vi "AIT 1553 - Parse RT Sysdef Tree Messages.vi"(8 "error in":errorcluster, 9 "RT_Messages":T1[](array[typedef]), 10 "Section Ptr":T3 format="%.0x") -> (0 "error out":errorcluster, 1 "RT_Messages Out":T1[](array[typedef]))   [LabVIEW 2013]
uses:
  <vilib>/NI Veristand/Custom Device API/Custom Device Item Ref.ctl
  Controls/1553_RT_Message.ctl
  Controls/664 -Param.ctl
  Controls and Global/Global.vi
  <vilib>/NI Veristand/Custom Device Tools/Custom Device Utility Library/NI VeriStand - Search for Item by Name.vi
  <vilib>/NI Veristand/Custom Device API/Get Item Property (I32).vi
  <vilib>/NI Veristand/Custom Device API/Get Item Property (Double).vi
  <vilib>/NI Veristand/Custom Device API/Get Item Property (Boolean).vi
  AIT 664 Custom Device.lvlib
  <vilib>/NI Veristand/Custom Device Tools/Custom Device Utility Library/Custom Device Utility Library.lvlib
  <vilib>/NI Veristand/Custom Device API/Custom Device API.lvlib
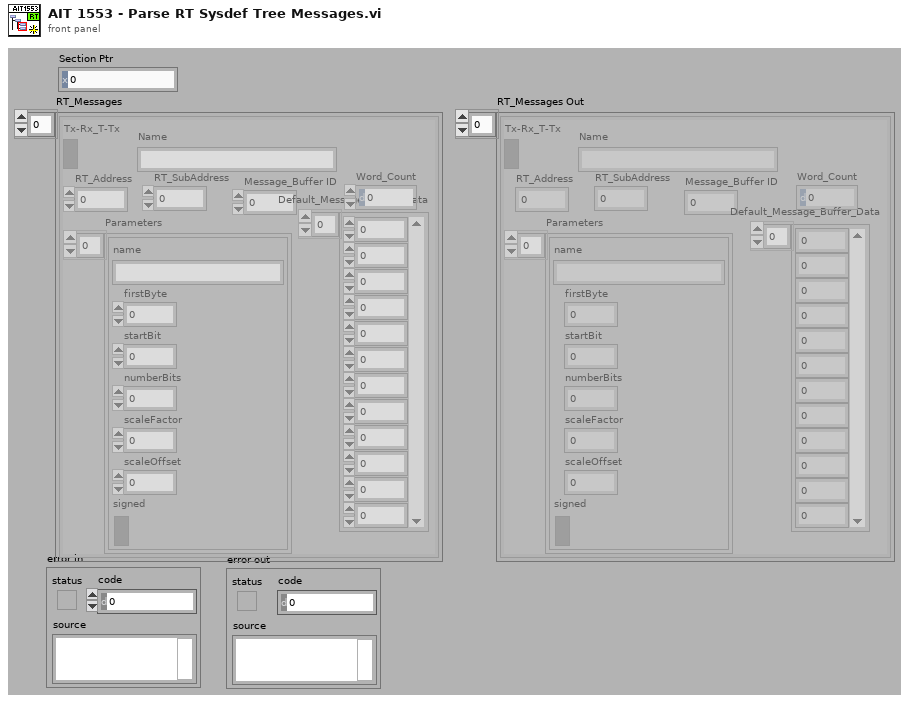
[diagram p1: front panel]
types:
  T1 = typedef "AIT 664 Custom Device.lvlib/1553_RT_Message.ctl" = cluster{"RT_Address":u8, "RT_SubAddress":u8, "Tx-Rx_T-Tx":bool, "Parameters":T2[], "Message_Buffer ID":u16, "Default_Message_Buffer_Data":u16[], "Word_Count":u8, "Name":string}
  T2 = typedef "AIT 664 Custom Device.lvlib/664 -Param.ctl" = cluster{"name":string, "firstByte":i32, "startBit":i32, "numberBits":i32, "scaleFactor":dbl, "scaleOffset":dbl, "signed":bool}
  T3 = typedef "Custom Device API.lvlib/Custom Device Item Ref.ctl" = u64
  T4 = typedef "Custom Device API.lvlib/Custom Device Item Info.ctl" = cluster{"Name":string, "Is Channel":bool, "GUID":string, "Is Waveform":bool}
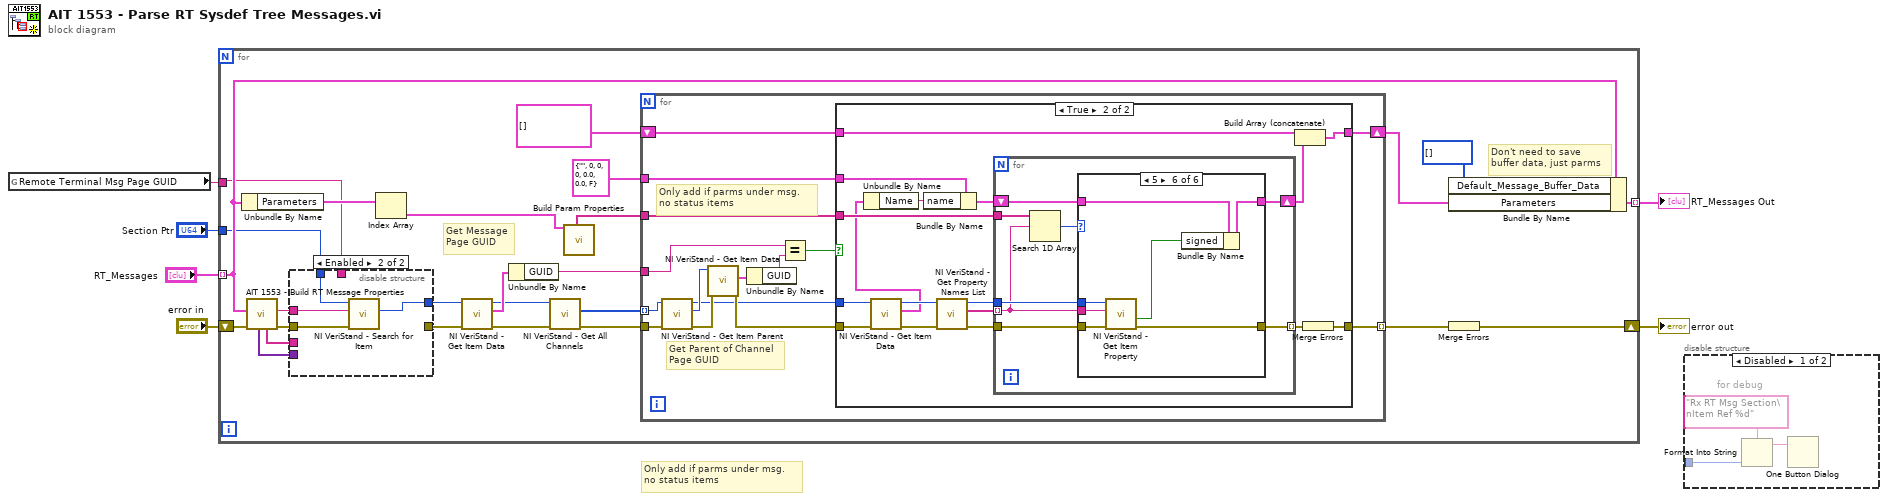
[diagram p0: block diagram]
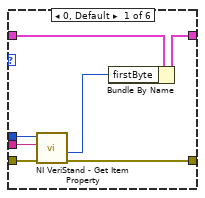
[diagram p4: hidden frame]
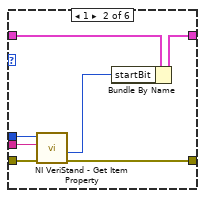
[diagram p5: hidden frame]
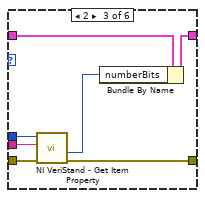
[diagram p6: hidden frame]
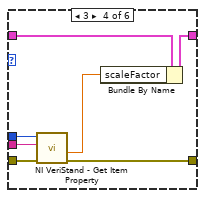
[diagram p7: hidden frame]
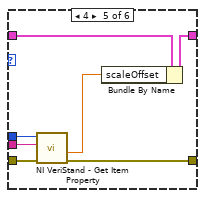
[diagram p8: hidden frame]
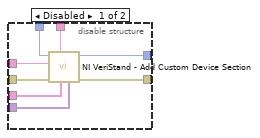
[diagram p9: hidden frame]
diagram:
  # "Only add if parms under msg.\nno status items"
  n1 = global read "Global.vi" "Remote Terminal Msg Page GUID"() -> (w3:string)
  n2 = for {
    shift-right: [w18] -> w6
    shift-left: "error in" -> [w32]
    tunnel: "Section Ptr" -> [w23]
    tunnel: "RT_Messages" -> [w25] mode=indexing
    tunnel: w3 -> [w24]
    tunnel: [w17] -> w1 mode=indexing
    # "Get Message\nPage GUID"
    # "Don't need to save\nbuffer data, just parms"
    n3 = Unbundle By Name(w25) -> ("Parameters"=w28:T2[])
    n4 = call "AIT 1553 - Build RT Message Properties.vi"("error in (no error)"=w32, "RT_Message"=w25) -> ("error out"=w21:errorcluster, "name"=w22:string, "Prop Names"=w20:string[], "Prop Values"=w19:variant[])  [unwired: 5 in, 1 out]
    n5 = disable-structure shown="Enabled" {
      disable-tunnel: w19 -> [w124 _]
      disable-tunnel: w20 -> [w123 _]
      disable-tunnel: w21 -> [w122 w127]
      disable-tunnel: w22 -> [w121 w128]
      disable-tunnel: w24 -> [w120 _]
      disable-tunnel: w23 -> [w119 w126]
      disable-tunnel: [w118 _] -> w13
      disable-tunnel: [w117 w125] -> w12
      frame Disabled {
        n6 = call <vilib>:"NI VeriStand - Add Custom Device Section.vi"("Property Values"=w124, "Property names"=w123, "GUID (Default Section)"=w120, "error in (no error)"=w122, "Section Name"=w121, "Parent Ref in"=w119) -> ("error out"=w118:errorcluster, "Section Ptr"=w117:T3)  [unwired: 2 in, 2 out]
      }
      frame Enabled {
        n7 = call-poly <vilib>:"NI VeriStand - Search for Item.vi"("error in"=w127, "Item Name"=w128, "Section Ref in"=w126) -> ("Item Ref"=w125:T3)  [unwired: 5 in, 3 out]
      }
    }
    n8 = Index Array(array=w28) -> (element=w29:T2)  [unwired: 1 in]
    n9 = call <vilib>:"NI VeriStand - Get Item Data.vi"("error in (no error)"=w13, "Item Ref in"=w12) -> ("error out"=w11:errorcluster, "Item Info"=w14:T4, "Item Ref out"=w10:T3)  [unwired: 6 in, 1 out]
    n10 = Unbundle By Name(w14) -> ("GUID"=w9:string)
    n11 = call <vilib>:"NI VeriStand - Get All Channels.vi"("error in"=w11, "Section Ref in"=w10) -> ("error out"=w26:errorcluster, "Channel Refs"=w27:T3[])  [unwired: 6 in, 2 out]
    n12 = call "Build Param Properties.vi"("Parameter"=w29) -> ("Prop Names"=w30:string[])  [unwired: 10 in, 8 out]
    n13 = for {
      tunnel: w26 -> [w41]
      tunnel: w27 -> [w42] mode=indexing
      tunnel: w30 -> [w47]
      tunnel: [w46] -> w31 mode=indexing
      tunnel: T2 {"name"="", "firstByte"=0, "startBit"=0, "numberBits"=0, "scaleFactor"=0.0, "scaleOffset"=0.0, "signed"=FALSE} ("1553 Parameter") -> [w45]
      tunnel: w9 -> [w37]
      shift-right: [w33] -> w7
      shift-left: T2[] [] -> [w34]
      # "Only add if parms under msg.\nno status items"
      # "Get Parent of Channel\nPage GUID"
      n14 = call <vilib>:"NI VeriStand - Get Item Parent.vi"("error in (no error)"=w41, "Item Ref in"=w42) -> ("error out"=w44:errorcluster, "Parent Ref"=w43:T3, "Item Ref out"=w39:T3)  [unwired: 6 in, 1 out]
      n15 = call <vilib>:"NI VeriStand - Get Item Data.vi"("error in (no error)"=w44, "Item Ref in"=w43) -> ("error out"=w40:errorcluster, "Item Info"=w38:T4)  [unwired: 6 in, 2 out]
      n16 = Unbundle By Name(w38) -> ("GUID"=w35:string)
      n17 = Equal?(x=w37, y=w35) -> (x = y?=w36:bool)
      n18 = case shown="True" w36 {
        tunnel: w47 -> [_ w64]
        tunnel: [w48 w61] -> w46
        tunnel: w45 -> [_ w57]
        tunnel: w40 -> [w48 w54]
        tunnel: w39 -> [_ w53]
        tunnel: w34 -> [w49 w52]
        tunnel: [w49 w50] -> w33
        frame False {
        }
        frame True {
          n19 = call <vilib>:"NI VeriStand - Get Item Data.vi"("error in (no error)"=w54, "Item Ref in"=w53) -> ("error out"=w60:errorcluster, "Item Info"=w55:T4, "Item Ref out"=w59:T3)  [unwired: 6 in, 1 out]
          n20 = Unbundle By Name(w55) -> ("Name"=w58:string)
          n21 = Bundle By Name(cluster=w57, "name"=w58) -> (w56:T2)
          n22 = call <vilib>:"NI VeriStand - Get Property Names List.vi"("error in (no error)"=w60, "Item Ref in"=w59) -> ("error out"=w66:errorcluster, "Property Names"=w65:string[], "Item Ref out"=w63:T3)  [unwired: 7 in]
          n23 = for {
            tunnel: w66 -> [w71]
            tunnel: w65 -> [w69] mode=indexing
            tunnel: w64 -> [w74]
            shift-right: [w68] -> w51
            shift-left: w56 -> [w72]
            tunnel: w63 -> [w70]
            tunnel: [w67] -> w62 mode=indexing
            n24 = Search 1D Array(1D array=w74, element=w69) -> (index of element=w73:i32)  [unwired: 1 in]
            n25 = case shown="5" w73 {
              tunnel: w72 -> [w81 w88 w95 w102 w109 w116]
              tunnel: w71 -> [w80 w87 w94 w101 w108 w115]
              tunnel: w70 -> [w79 w86 w93 w100 w107 w114]
              tunnel: w69 -> [w78 w85 w92 w99 w106 w113]
              tunnel: [w76 w83 w90 w97 w104 w111] -> w68
              tunnel: [w75 w82 w89 w96 w103 w110] -> w67
              frame 0, Default {
                n26 = call-poly <vilib>:"NI VeriStand - Get Item Property.vi"("error in (no error)"=w80, "Property Name"=w78, "Item Ref in"=w79) -> ("error out"=w75:errorcluster, "Value"=w77:i32)  [unwired: 5 in, 2 out]
                n27 = Bundle By Name(cluster=w81, "firstByte"=w77) -> (w76:T2)
              }
              frame 1 {
                n28 = call-poly <vilib>:"NI VeriStand - Get Item Property.vi"("error in (no error)"=w87, "Property Name"=w85, "Item Ref in"=w86) -> ("error out"=w82:errorcluster, "Value"=w84:i32)  [unwired: 5 in, 2 out]
                n29 = Bundle By Name(cluster=w88, "startBit"=w84) -> (w83:T2)
              }
              frame 2 {
                n30 = call-poly <vilib>:"NI VeriStand - Get Item Property.vi"("error in (no error)"=w94, "Property Name"=w92, "Item Ref in"=w93) -> ("error out"=w89:errorcluster, "Value"=w91:i32)  [unwired: 5 in, 2 out]
                n31 = Bundle By Name(cluster=w95, "numberBits"=w91) -> (w90:T2)
              }
              frame 3 {
                n32 = call-poly <vilib>:"NI VeriStand - Get Item Property.vi"("error in (no error)"=w101, "Property Name"=w99, "Item Ref in"=w100) -> ("error out"=w96:errorcluster, "Value"=w98:dbl)  [unwired: 5 in, 2 out]
                n33 = Bundle By Name(cluster=w102, "scaleFactor"=w98) -> (w97:T2)
              }
              frame 4 {
                n34 = call-poly <vilib>:"NI VeriStand - Get Item Property.vi"("error in (no error)"=w108, "Property Name"=w106, "Item Ref in"=w107) -> ("error out"=w103:errorcluster, "Value"=w105:dbl)  [unwired: 5 in, 2 out]
                n35 = Bundle By Name(cluster=w109, "scaleOffset"=w105) -> (w104:T2)
              }
              frame 5 {
                n36 = call-poly <vilib>:"NI VeriStand - Get Item Property.vi"("error in (no error)"=w115, "Property Name"=w113, "Item Ref in"=w114) -> ("error out"=w110:errorcluster, "Value"=w112:bool)  [unwired: 5 in, 2 out]
                n37 = Bundle By Name(cluster=w116, "signed"=w112) -> (w111:T2)
              }
            }
          }
          n38 = Build Array (concatenate)(w52, w51) -> (w50:T2[])
          n39 = Merge Errors(w62) -> (w61:errorcluster)
        }
      }
    }
    n40 = Bundle By Name(cluster=w25, "Default_Message_Buffer_Data"=u16[] [], "Parameters"=w7) -> (w17:T1)
    n41 = Merge Errors(w31) -> (w18:errorcluster)
  }
  "error out" <- w6
  "RT_Messages Out" <- w1
  n42 = disable-structure shown="Disabled" {
    disable-tunnel: _ -> [w129 _]
    frame Disabled {
      # "for debug"
      n43 = Format Into String(format string="Rx RT Msg Section\nItem Ref %d" ("message"), w129) -> (resulting string=w131:string)  [unwired: 2 in, 1 out]
      n44 = One Button Dialog(message=w131) -> ()  [unwired: 1 in, 1 out]
    }
    frame Enabled {
    }
  }
